vi "getRef.vi"(8 "error in (no error)":errorcluster) -> (0 "error out":errorcluster, 2 "items_controller_ref":refnum<class "Items Controller.lvclass">)   [LabVIEW 2015, in "Items Controller.lvclass"]
uses:
  Items Controller.lvclass
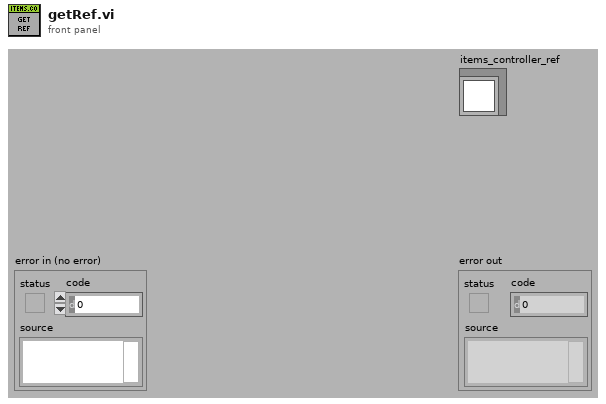
[diagram p1: front panel]
types:
  T1 = typedef "Items Controller.lvclass/ClassAttributesRef.ctl" = refnum<data-value>
  T2 = typedef "Items Controller.lvclass/ClassAttributes.ctl" = cluster{"Dummy":bool, "items_controller_ref":refnum<class "Items Controller.lvclass">}
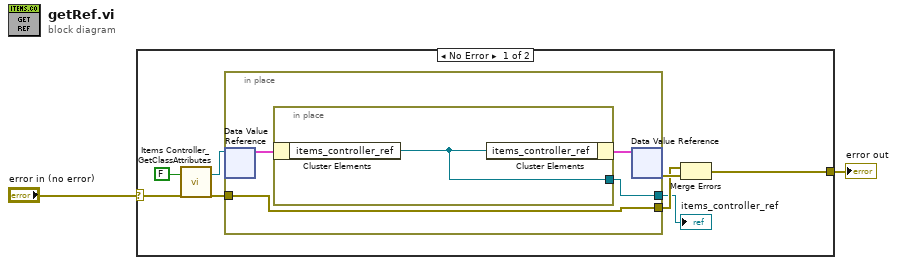
[diagram p0: block diagram]
diagram:
  n1 = case shown="No Error" "error in (no error)" {
    selector: "error in (no error)" -> [w6 w16]
    tunnel: [w10 w16] -> w1
    frame No Error {
      n2 = call "Items Controller_GetClassAttributes.vi"("return data? (T)"=FALSE, "error in (no error)"=w6) -> ("class attributes ref"=w4:T1, "error out"=w5:errorcluster)  [unwired: 14 in, 2 out]
      n3 = in-place {
        in-place-border: w5 -> [w12]
        in-place-border: [w12] -> w8
        in-place-border: [w11] -> w3
        n4 = in-place-dvr #1(w4) -> (w13:T2)  [unwired: 1 out]
        n5 = in-place {
          in-place-border: [w15] -> w11
          n6 = in-place-cluster #2(w13) -> ("items_controller_ref"=w15:refnum<class "Items Controller.lvclass">)
          n7 = in-place-cluster #2("items_controller_ref"=w15) -> (w14:T2)
        }
        n8 = in-place-dvr #1(w14) -> (w9:errorcluster)  [unwired: 1 out]
      }
      "items_controller_ref" <- w3
      n9 = Merge Errors(w8, w9) -> (w10:errorcluster)
    }
    frame Error {
    }
  }
  "error out" <- w1
